vi "ma_sml_FFT Size and RBW (RT Zoom).vi"(0 "window":u16(ring) items=["Rectangle"=0, "Hanning"=1, "Hamming"=2, "Blackman-Harris"=3, "Exact Blackman"=4, "Blackman"=5, "Flat Top"=6, "4 Term B-Harris "=7, "7 Term B-Harris"=8, "Low Sidelobe"=9, "Blackman Nuttall"=11, "Triangle"=30, "Bartlett-Hanning"=31, "Bohman"=32, "Parzen"=33, "Welch"=34, "Kaiser"=60, "Dolph-Chebyshev"=61, "Gaussian"=62], 1 "RBW definition":enum16{"3dB", "6dB", "ENBW", "bin width"}(ring), 5 "RBW":dbl format="%.2f", 7 "zoom":dbl format="%.7f", 9 "spectral lines":i32=-1, 11 "fs":dbl format="%.2f", 12 "input signal type":enum16{"real", "complex modulated"}(ring)) -> (2 "RBW actual":dbl format="%.2f", 3 "span":dbl format="%.2f", 4 "block size":i32=-1, 6 "trim":dbl format="%.5f", 8 "window size":i32=-1, 10 "spectral lines actual":i32=-1, 14 "zoom factor":i32=-1, 15 "FFT Size":i32=-1)   [LabVIEW 2020, in "NI_MAPro.lvlib"]
uses:
  NI_MAPro.lvlib
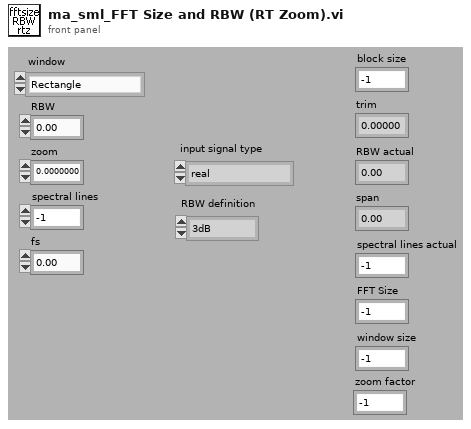
[diagram p1: front panel]
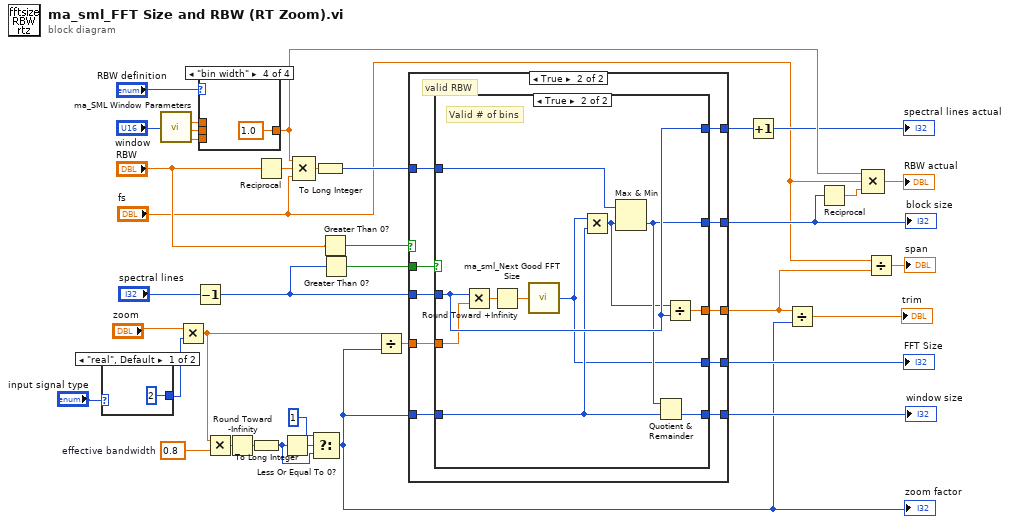
[diagram p0: block diagram]
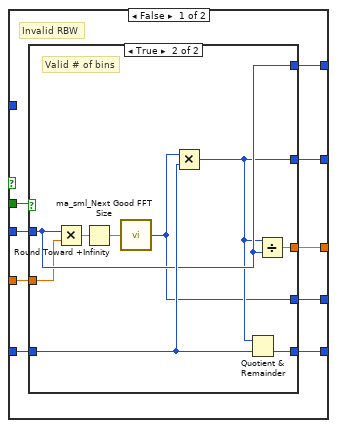
[diagram p5: hidden frame]
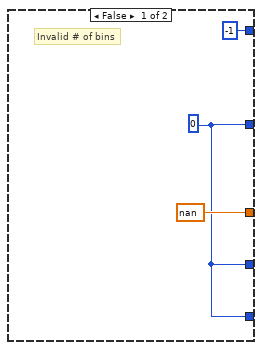
[diagram p6: hidden frame]
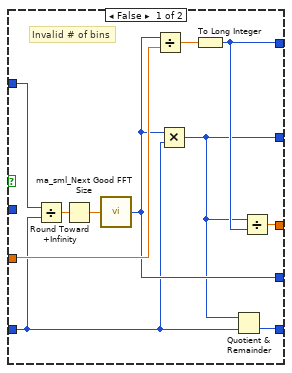
[diagram p7: hidden frame]
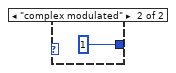
[diagram p8: hidden frame]
diagram:
  w16 = 0.8  # effective bandwidth
  n1 = case shown="\"real\", Default" "input signal type" {
    tunnel: [2 1] -> w9
    frame "real", Default {
    }
    frame "complex modulated" {
    }
  }
  n2 = call "ma_SML Window Parameters.vi"("window"="window") -> ("ENBW"=w20:dbl, "3dB BW"=w19:dbl, "6dB BW"=w18:dbl)  [unwired: 1 out]
  n3 = Multiply(x="zoom", y=w9) -> (x*y=w10:dbl)
  n4 = Decrement(x="spectral lines") -> (x-1=w3:i32)
  n5 = case shown="\"bin width\"" "RBW definition" {
    tunnel: w20 -> [_ _ w42 _]
    tunnel: w19 -> [w40 _ _ _]
    tunnel: w18 -> [_ w41 _ _]
    tunnel: [w40 w41 w42 1.0 ("ENBW")] -> w21
    frame "3dB", Default {
    }
    frame "6dB" {
    }
    frame "ENBW" {
    }
    frame "bin width" {
    }
  }
  n6 = Multiply(x=w10, y=w16) -> (x*y=w13:dbl)
  n7 = Round Toward -Infinity(1:w13) -> (0:w14:dbl)
  n8 = To Long Integer(number=w14) -> (32bit integer=w5:i32)
  n9 = Reciprocal(x="RBW") -> (1/x=w36:dbl)
  n10 = Less Or Equal To 0?(x=w5) -> (x <= 0?=w7:bool)
  n11 = Compound Arithmetic op=MULTIPLY(w21, w36, "fs") -> (w35:dbl)
  n12 = Select(t=1, s=w7, f=w5) -> (s? t:f=w6:i32)
  "zoom factor" <- w6
  n13 = To Long Integer(number=w35) -> (32bit integer=w34:i32)
  n14 = Greater Than 0?(x="RBW") -> (x > 0?=w30:bool)
  n15 = Greater Than 0?(x=w3) -> (x > 0?=w32:bool)
  n16 = Divide(x=w10, y=w6) -> (x/y=w15:dbl)
  n17 = case shown="True" w30 {
    tunnel: w34 -> [_ w74]
    tunnel: [w51 w71] -> w8
    tunnel: [w52 w73] -> w26
    tunnel: w3 -> [w46 w72]
    tunnel: w32 -> [w50 w70]
    tunnel: w6 -> [w45 w69]
    tunnel: [w49 w68] -> w25
    tunnel: [w47 w67] -> w28
    tunnel: [w48 w66] -> w27
    tunnel: w15 -> [w44 w65]
    frame False {
      # "Invalid RBW"
      n18 = case shown="True" w50 {
        tunnel: [-1 w61] -> w52
        tunnel: [nan w57] -> w51
        tunnel: [w54 w60] -> w49
        tunnel: [w54 w59] -> w48
        tunnel: [w54 w58] -> w47
        tunnel: w46 -> [_ w61]
        tunnel: w45 -> [_ w62]
        tunnel: w44 -> [_ w56]
        frame False {
          w54 = 0
          # "Invalid # of bins"
        }
        frame True {
          # "Valid # of bins"
          n19 = Multiply(x=w61, y=w56) -> (x*y=w63:dbl)
          n20 = Round Toward +Infinity(x=w63) -> (ceil(x): smallest int >= x=w64:dbl)
          n21 = call "ma_sml_Next Good FFT Size.vi"("FFT Size"=w64) -> ("least bigger good size"=w59:i32)
          n22 = Multiply(x=w59, y=w62) -> (x*y=w60:i32)
          n23 = Quotient & Remainder(x=w60, y=w62) -> (floor(x/y)=w58:i32)  [unwired: 1 out]
          n24 = Divide(x=w60, y=w61) -> (x/y=w57:dbl)
        }
      }
    }
    frame True {
      # "valid RBW"
      n25 = case shown="True" w70 {
        tunnel: w74 -> [w83 w90]
        tunnel: [w77 w93] -> w73
        tunnel: w72 -> [_ w93]
        tunnel: [w80 w94] -> w71
        tunnel: w69 -> [w75 w92]
        tunnel: [w76 w89] -> w68
        tunnel: [w78 w91] -> w67
        tunnel: [w79 w87] -> w66
        tunnel: w65 -> [w82 w88]
        frame False {
          # "Invalid # of bins"
          n26 = Divide(x=w83, y=w75) -> (x/y=w85:dbl)
          n27 = Round Toward +Infinity(x=w85) -> (ceil(x): smallest int >= x=w84:dbl)
          n28 = call "ma_sml_Next Good FFT Size.vi"("FFT Size"=w84) -> ("least bigger good size"=w79:i32)
          n29 = Divide(x=w79, y=w82) -> (x/y=w81:dbl)
          n30 = Multiply(x=w79, y=w75) -> (x*y=w76:i32)
          n31 = To Long Integer(number=w81) -> (32bit integer=w77:i32)
          n32 = Quotient & Remainder(x=w76, y=w75) -> (floor(x/y)=w78:i32)  [unwired: 1 out]
          n33 = Divide(x=w76, y=w77) -> (x/y=w80:dbl)
        }
        frame True {
          # "Valid # of bins"
          n34 = Multiply(x=w93, y=w88) -> (x*y=w96:dbl)
          n35 = Round Toward +Infinity(x=w96) -> (ceil(x): smallest int >= x=w95:dbl)
          n36 = call "ma_sml_Next Good FFT Size.vi"("FFT Size"=w95) -> ("least bigger good size"=w87:i32)
          n37 = Multiply(x=w87, y=w92) -> (x*y=w86:i32)
          n38 = Max & Min(x=w90, y=w86) -> (min(x,y)=w89:i32)  [unwired: 1 out]
          n39 = Quotient & Remainder(x=w89, y=w92) -> (floor(x/y)=w91:i32)  [unwired: 1 out]
          n40 = Divide(x=w86, y=w93) -> (x/y=w94:dbl)
        }
      }
    }
  }
  "block size" <- w25
  "FFT Size" <- w27
  "window size" <- w28
  n41 = Increment(x=w26) -> (x+1=→"spectral lines actual":i32)
  n42 = Divide(x=w8, y=w6) -> (x/y=→"trim":dbl)
  n43 = Reciprocal(x=w25) -> (1/x=w24:dbl)
  n44 = Compound Arithmetic op=MULTIPLY(w21, "fs", w24) -> (→"RBW actual":dbl)
  n45 = Divide(x="fs", y=w8) -> (x/y=→"span":dbl)
